vi "Create.vi"(8 "error in (no error)":errorcluster) -> (0 "error out":errorcluster, 3 "Execution UI Out":refnum<class "Execution UI.lvclass">)   [LabVIEW 2020, in "Execution UI.lvclass"]
uses:
  Execution UI.lvclass
  Execution UI.lvclass/Execution UI.ctl
  Result Model/Result Model.lvclass
  Configuration Manager/UI Configuration Manager.lvclass
  Private/TypeDefs/Message Cluster.ctl
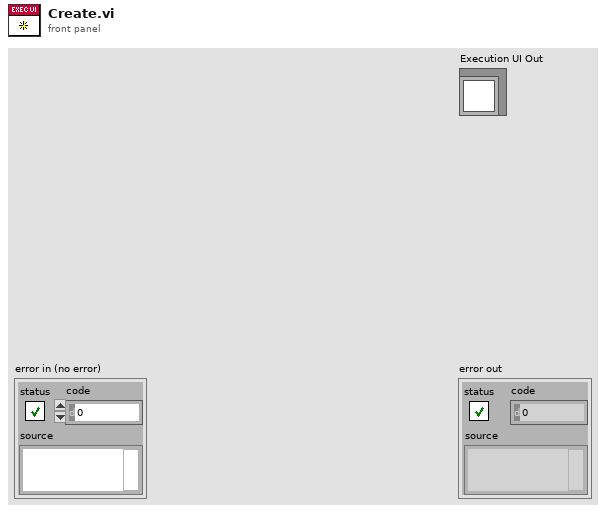
[diagram p1: front panel]
types:
  T1 = typedef "Execution UI.lvclass/Message Cluster.ctl" = cluster{"Message":string, "Message Data":variant}
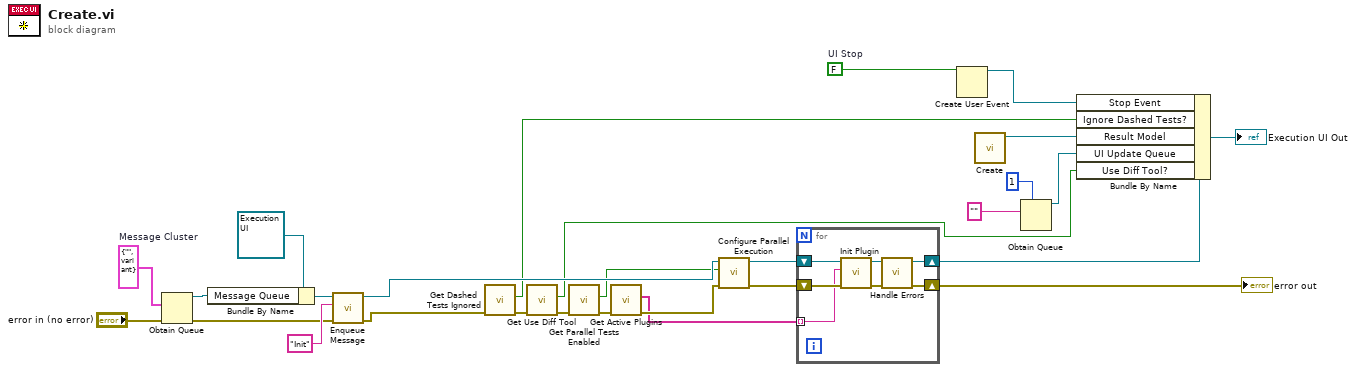
[diagram p0: block diagram]
diagram:
  w5 = T1 {"Message"="", "Message Data"=variant}  # Message Cluster
  w25 = FALSE  # UI Stop
  n1 = Obtain Queue(element data type=w5, error in (no error)="error in (no error)") -> (queue out=w2:refnum<queue>, error out=w3:errorcluster)  [unwired: 3 in, 1 out]
  n2 = Bundle By Name(cluster=refnum<class "Execution UI.lvclass"> refnum ("Execution UI In"), "Message Queue"=w2) -> (w1:refnum<class "Execution UI.lvclass">)
  n3 = call "Enqueue Message.vi"("error in (no error)"=w3, "Message"="Init", "Process In"=w1) -> ("error out"=w18:errorcluster, "Process Out"=w17:refnum<class "Execution UI.lvclass">)  [unwired: 7 in]
  n4 = call "Get Dashed Tests Ignored.vi"("error in (no error)"=w18) -> ("error out"=w8:errorcluster, "Ignore Dashed?"=w9:bool)  [unwired: 9 in]
  n5 = call "Get Use Diff Tool.vi"("error in (no error)"=w8) -> ("error out"=w7:errorcluster, "Diff in Descriptions?"=w6:bool)  [unwired: 9 in]
  n6 = call "Get Parallel Tests Enabled.vi"("error in (no error)"=w7) -> ("error out"=w19:errorcluster, "Parallel tetss enabled?"=w16:bool)  [unwired: 9 in]
  n7 = call "Get Active Plugins.vi"("error in (no error)"=w19) -> ("error out"=w15:errorcluster, "Plugins"=w14:string[])  [unwired: 9 in]
  n8 = call "Configure Parallel Execution.vi"("error in (no error)"=w15, "Enable Parallel Execution?"=w16, "Execution UI In"=w17) -> ("error out"=w13:errorcluster, "Execution UI Out"=w11:refnum<class "Execution UI.lvclass">)  [unwired: 7 in]
  n9 = for {
    tunnel: w14 -> [w31] mode=indexing
    shift-right: [w29] -> w12
    shift-left: w13 -> [w34]
    shift-right: [w32] -> w10
    shift-left: w11 -> [w33]
    n10 = call "Init Plugin.vi"("error in (no error)"=w34, "Plugin"=w31, "Execution UI in"=w33) -> ("error out"=w30:errorcluster, "Execution UI out"=w32:refnum<class "Execution UI.lvclass">)  [unwired: 7 in]
    n11 = call "Handle Errors.vi"("error in (no error)"=w30) -> ("error out"=w29:errorcluster)  [unwired: 10 in]
  }
  "error out" <- w12
  n12 = Create User Event(user event datatype=w25) -> (user event=w24:refnum<user-event>)  [unwired: 1 in, 1 out]
  n13 = call "Create.vi"() -> ("Result Model out"=w20:refnum<class "Result Model.lvclass">)  [unwired: 10 in, 1 out]
  n14 = Obtain Queue(max queue size (-1, unlimited)=1, element data type="") -> (queue out=w21:refnum<queue>)  [unwired: 3 in, 2 out]
  n15 = Bundle By Name(cluster=w10, "Stop Event"=w24, "Ignore Dashed Tests?"=w9, "Result Model"=w20, "UI Update Queue"=w21, "Use Diff Tool?"=w6) -> (→"Execution UI Out":refnum<class "Execution UI.lvclass">)
